vi "DWF MSO Configure Advanced Digital Timing.vi"(0 "Instrument Handle In":u32, 5 "Digital Sample Rate Control":i32(ring) items=["Automatic", "Manual"], 7 "Digital Sample Rate":dbl=100000.0, 9 "Buffer Control":i32(ring) items=["Automatic", "Manual"], 11 "Error In":errorcluster caption="Error In (no error)", 12 "Buffer Pretrigger Percent":dbl=50.0) -> (4 "Instrument Handle Out":u32, 15 "Error Out":errorcluster)   [LabVIEW 2015, in "DigilentWF.lvlib"]
doc: "Configures the rate and buffer settings of the logic analyzer. This VI allows for more advanced configuration options than <B>MSO Configure Timing.</B>"
uses:
  <vilib>/DigilentWF/DigilentWF.lvlib
  dwf.dll
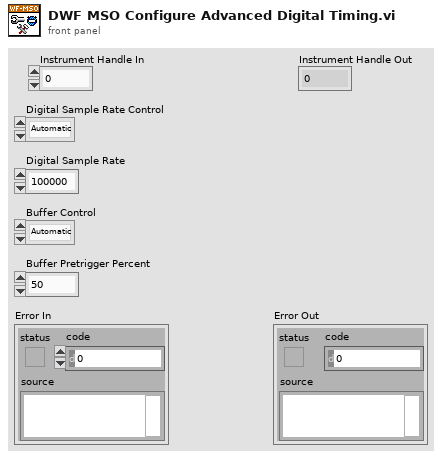
[diagram p1: front panel]
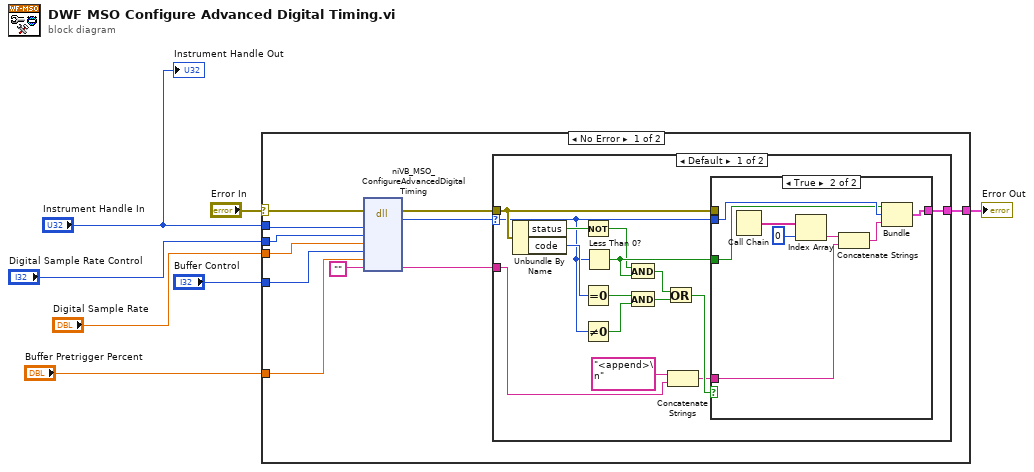
[diagram p0: block diagram]
diagram:
  n1 = case "outter_case" shown="No Error" "Error In" {
    selector: "Error In" -> [w17 w44]
    tunnel: [w18 w44] -> w6
    tunnel: "Instrument Handle In" -> [w16 _]
    tunnel: "Digital Sample Rate Control" -> [w15 _]
    tunnel: "Digital Sample Rate" -> [w14 _]
    tunnel: "Buffer Control" -> [w13 _]
    tunnel: "Buffer Pretrigger Percent" -> [w12 _]
    frame No Error {
      n2 = dll-call lib="dwf.*" fn="niVB_MSO_ConfigureAdvancedDigitalTiming"(error in=w17, "instrumentHandle"=w16, "digitalSampleRateControl"=w15, "digitalSampleRate"=w14, "bufferControl"=w13, "bufferPretriggerPercent"=w12, "szError"="") -> (error out=w11:errorcluster, "return type"=w10:u32, "szError"=w8:string)  [unwired: 7 in, 1 out]
      n3 = case "inner_case" shown="Default" w10 {
        selector: w10 -> [w23 _]
        tunnel: w11 -> [w24 w43]
        tunnel: [w20 w43] -> w18
        tunnel: w8 -> [w19 _]
        frame Default {
          n4 = Unbundle By Name(w24) -> ("status"=w28:bool, "code"=w32:i32)
          n5 = Not(x=w28) -> (.not. x?=w31:bool)
          n6 = Equal To 0?(x=w32) -> (x = 0?=w27:bool)
          n7 = Not Equal To 0?(x=w23) -> (x != 0?=w30:bool)
          n8 = Less Than 0?(x=w23) -> (x < 0?=w33:bool)
          n9 = And(x=w31, y=w33) -> (x .and. y?=w29:bool)
          n10 = And(x=w27, y=w30) -> (x .and. y?=w26:bool)
          n11 = Or(x=w29, y=w26) -> (x .or. y?=w25:bool)
          n12 = Concatenate Strings("<append>\n" ("string"), w19) -> (w22:string)
          n13 = case shown="True" w25 {
            tunnel: [w34 w41] -> w20
            tunnel: w23 -> [_ w40]
            tunnel: w33 -> [_ w39]
            tunnel: w24 -> [w34 _]
            tunnel: w22 -> [_ w35]
            frame False {
            }
            frame True {
              n14 = Call Chain() -> (call chain=w38:string[])
              n15 = Index Array(array=w38, index=0) -> (element=w37:string)
              n16 = Concatenate Strings(w37, w35) -> (w42:string)
              n17 = Bundle(w39, "return type"=w40, w42) -> (w41:cluster{bool, "return type":u32, string})  [unwired: 1 out]
            }
          }
        }
        frame 0 {
        }
      }
    }
    frame Error {
    }
  }
  "Error Out" <- w6
  "Instrument Handle Out" <- "Instrument Handle In"
